vi "day 8 task 1.vi"() -> ()   [LabVIEW 2019]
panel:
  out "x > 0?":bool[][](array[boolean])
  out "Array 2":u8[][](array[numeric])
  out "sum":i16
  out "Array":bool[][][](array[boolean])
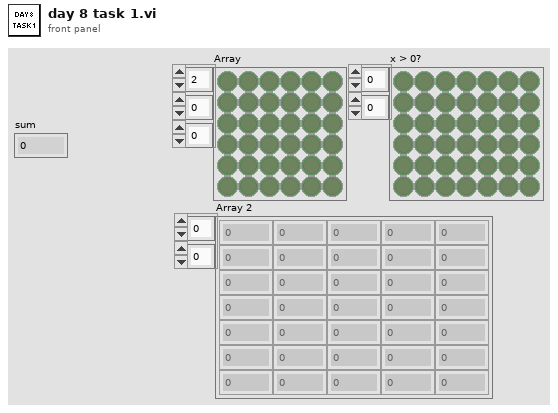
[diagram p1: front panel]
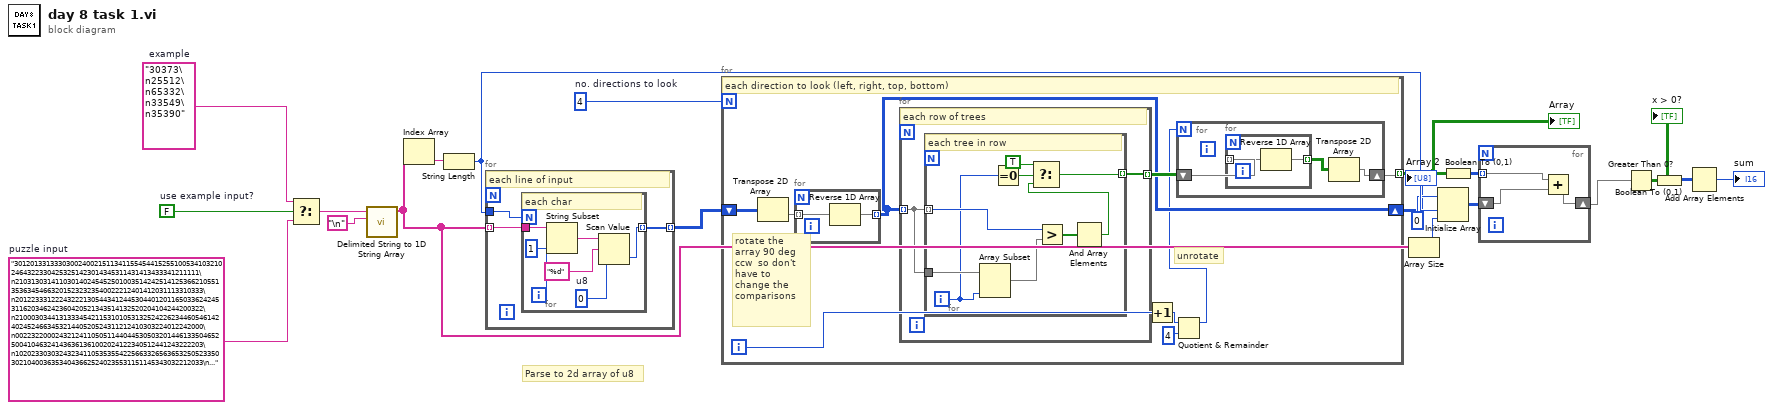
[diagram p0: block diagram]
diagram:
  w15 = 4  # no. directions to look
  w18 = "30373\n25512\n65332\n33549\n35390"  # example
  w19 = FALSE  # use example input?
  w20 = "301201331333030024002151134115545441525510053410321024643223304253251423014345311431413433341211111\n210313031411030140245452501003514242514125366210551353634546632015232323540022212401412031113310333\n201223331222432221305443412445304401201165033624245311620346242360420521343514132520204104244200322\n210003034413133345421153101053132524226234460546142402452466345321440520524311212410303224012242000\n002232200024321241105051144044530503201446133504652500410463241436361361002024122340512441243222203\n102023303032432341105353554225663326563653250523350302104003635340436625240235531151145343032212033\n..."  # puzzle input
  # "Parse to 2d array of u8"
  n1 = Select(t=w18, s=w19, f=w20) -> (s? t:f=w17:string)
  n2 = call <vilib>:"Delimited String to 1D String Array.vi"("delimiter"="\n", "delimited string"=w17) -> ("string array"=w7:string[])  [unwired: 9 in]
  n3 = Index Array(array=w7) -> (element=w14:string)  [unwired: 1 in]
  n4 = String Length(string=w14) -> (length=w9:i32)
  n5 = for {
    tunnel: w7 -> [w23] mode=indexing
    tunnel: [w22] -> w13 mode=indexing
    tunnel: w9 -> [w21]
    # "each line of input"
    n6 = for {
      N: w21 -> [_]
      tunnel: w23 -> [w30]
      tunnel: [w26] -> w22 mode=indexing
      i -> [w24]
      w27 = u8 0  # u8
      # "each char"
      n7 = String Subset(string=w30, offset (0)=w24, length (rest)=1 ("length (rest)")) -> (substring=w29:string)
      n8 = Scan Value(string=w29, format string="%d", default (0 dbl)=w27) -> (value=w26:u8)  [unwired: 1 out]
    }
  }
  n9 = for {
    N: w15 -> [_]
    shift-right: [w35] -> w1
    shift-left: w13 -> [w39]
    tunnel: [w38] -> w11 mode=indexing
    i -> [w32]
    # "unrotate"
    # "rotate the array 90 deg ccw  so don't have to change the comparisons"
    # "each direction to look (left, right, top, bottom)"
    n10 = Transpose 2D Array(2D array=w39) -> (transposed array=w36:u8[][])
    n11 = for {
      tunnel: w36 -> [w41] mode=indexing
      tunnel: [w40] -> w35 mode=indexing
      n12 = Reverse 1D Array(array=w41) -> (reversed array=w40:u8[])
    }
    n13 = for {
      tunnel: w35 -> [w48] mode=indexing
      tunnel: [w47] -> w37 mode=indexing
      # "each row of trees"
      n14 = for {
        tunnel: w48 -> [w57] mode=indexing
        tunnel: w48 -> [w56]
        tunnel: [w49] -> w47 mode=indexing
        i -> [w54]
        # "each tree in row"
        n15 = Array Subset(array=w56, length=w54) -> (w55:u8[])  [unwired: 1 in]
        n16 = Equal To 0?(x=w54) -> (x = 0?=w53:bool)
        n17 = Greater?(x=w57, y=w55) -> (0:w51:bool[])
        n18 = And Array Elements(Boolean array=w51) -> (logical AND=w50:bool)
        n19 = Select(t=TRUE, s=w53, f=w50) -> (s? t:f=w49:bool)
      }
    }
    n20 = Increment(x=w32) -> (x+1=w33:i32)
    n21 = Quotient & Remainder(x=w33, y=4) -> (x-y*floor(x/y)=w31:i32)  [unwired: 1 out]
    n22 = for {
      N: w31 -> [_]
      shift-right: [w42] -> w38
      shift-left: w37 -> [w44]
      n23 = for {
        tunnel: w44 -> [w46] mode=indexing
        tunnel: [w45] -> w43 mode=indexing
        n24 = Reverse 1D Array(array=w46) -> (reversed array=w45:bool[])
      }
      n25 = Transpose 2D Array(2D array=w43) -> (transposed array=w42:bool[][])
    }
  }
  "Array" <- w11
  "Array 2" <- w1
  n26 = Array Size(array=w7) -> (size(s)=w8:i32)
  n27 = Initialize Array(i16 0, w9, w8) -> (w6:i16[][])
  n28 = Boolean To (0,1)(Boolean=w11) -> (0, 1=w10:i16[][][])
  n29 = for {
    tunnel: w10 -> [w59] mode=indexing
    shift-right: [w60] -> w4
    shift-left: w6 -> [w58]
    n30 = Add(x=w59, y=w58) -> (x+y=w60:i16[][])
  }
  n31 = Greater Than 0?(x=w4) -> (x > 0?=w2:bool[][])
  "x > 0?" <- w2
  n32 = Boolean To (0,1)(Boolean=w2) -> (0, 1=w3:i16[][])
  n33 = Add Array Elements(numeric array=w3) -> (sum=→"sum":i16)
